vi "Generate CW RF.vi"(8 "error in (no error)":errorcluster, 11 "resource name":refnum<k15>) -> (0 "error out":errorcluster)   [LabVIEW 2018]
panel:
  in  "power level (dBm)":dbl=-90.0 format="%.2f"
  in  "frequency (Hz)":dbl=100000000.0 format="%.2p"
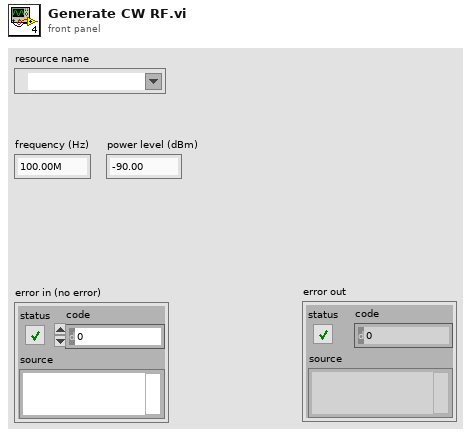
[diagram p1: front panel]
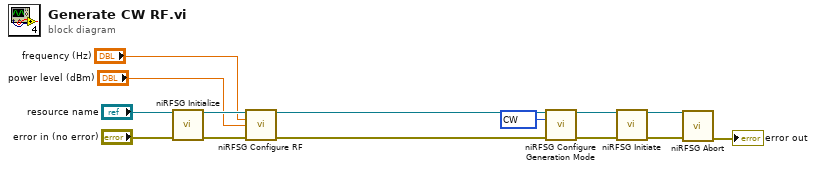
[diagram p0: block diagram]
diagram:
  w3 = 1000 items=["CW"=1000, "Arb Waveform"=1001, "Script"=1002] ("generation mode")
  n1 = call <instrlib>:"niRFSG Initialize.vi"("resource name"="resource name", "error in"="error in (no error)") -> ("instrument handle"=w11:refnum<k15>, "error out"=w10:errorcluster)  [unwired: 12 in]
  n2 = call <instrlib>:"niRFSG Configure RF.vi"("instrument handle"=w11, "frequency (Hz)"="frequency (Hz)", "power level (dBm)"="power level (dBm)", "error in"=w10) -> ("instrument handle out"=w1:refnum<k15>, "error out"=w2:errorcluster)  [unwired: 10 in]
  n3 = call <instrlib>:"niRFSG Configure Generation Mode.vi"("instrument handle"=w1, "generation mode"=w3, "error in"=w2) -> ("instrument handle out"=w9:refnum<k15>, "error out"=w8:errorcluster)  [unwired: 11 in]
  n4 = call <instrlib>:"niRFSG Initiate.vi"("instrument handle"=w9, "error in"=w8) -> ("instrument handle out"=w7:refnum<k15>, "error out"=w6:errorcluster)  [unwired: 12 in]
  n5 = call <instrlib>:"niRFSG Abort.vi"("instrument handle"=w7, "error in"=w6) -> ("error out"=→"error out":errorcluster)  [unwired: 12 in, 1 out]
